vi "Signal1.vi"(10 "Iteration":i32) -> (0 "Stop Loop":bool, 2 "Output":dbl)   [LabVIEW 2019]
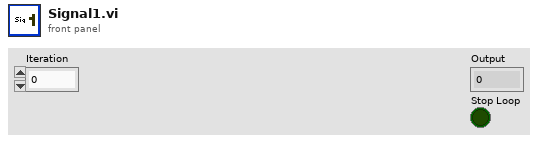
[diagram p1: front panel]
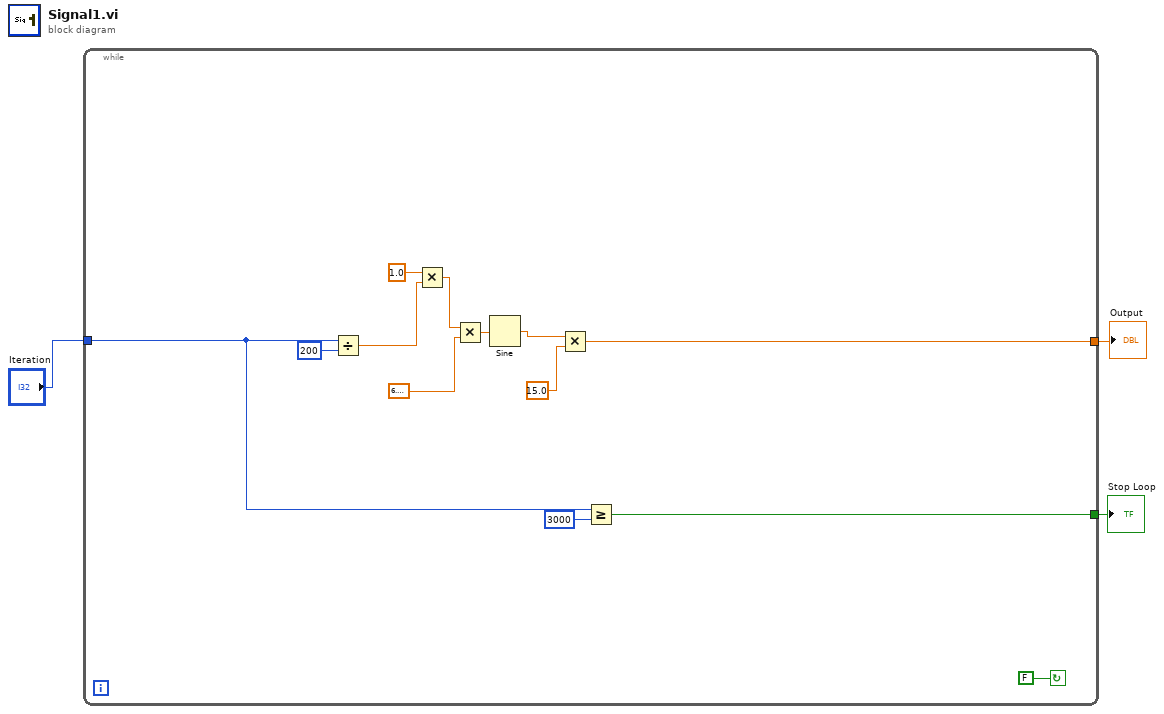
[diagram p0: block diagram]
diagram:
  n1 = while {
    tunnel: "Iteration" -> [w9]
    tunnel: [w10] -> w2
    tunnel: [w7] -> w1
    stop <- FALSE continue-if-true
    n2 = Divide(x=w9, y=200) -> (x/y=w14:dbl)
    n3 = Multiply(x=1.0, y=w14) -> (x*y=w5:dbl)
    n4 = Multiply(x=w5, y=6.283185307179586) -> (x*y=w6:dbl)
    n5 = Sine(x=w6) -> (sin(x)=w12:dbl)
    n6 = Multiply(x=w12, y=15.0) -> (x*y=w10:dbl)
    n7 = Greater Or Equal?(x=w9, y=3000) -> (x >= y?=w7:bool)
  }
  "Output" <- w2
  "Stop Loop" <- w1
